vi "VisualInspection.vi"(0 "Picture Name":string, 1 "Upper":dbl, 2 "Lower":dbl, 5 "MessageIn":string) -> (3 "Message:":string, 7 "Result":string, 9 "Next Step STS":bool, 10 "Button Pressing Status":string)   [LabVIEW 2011]
panel:
  out "appended path":path
  out "LED Pressing Status":string
  in  "No Light Up On LED":bool
  in  "Light Up on LED":bool
  out "Picture:":picture
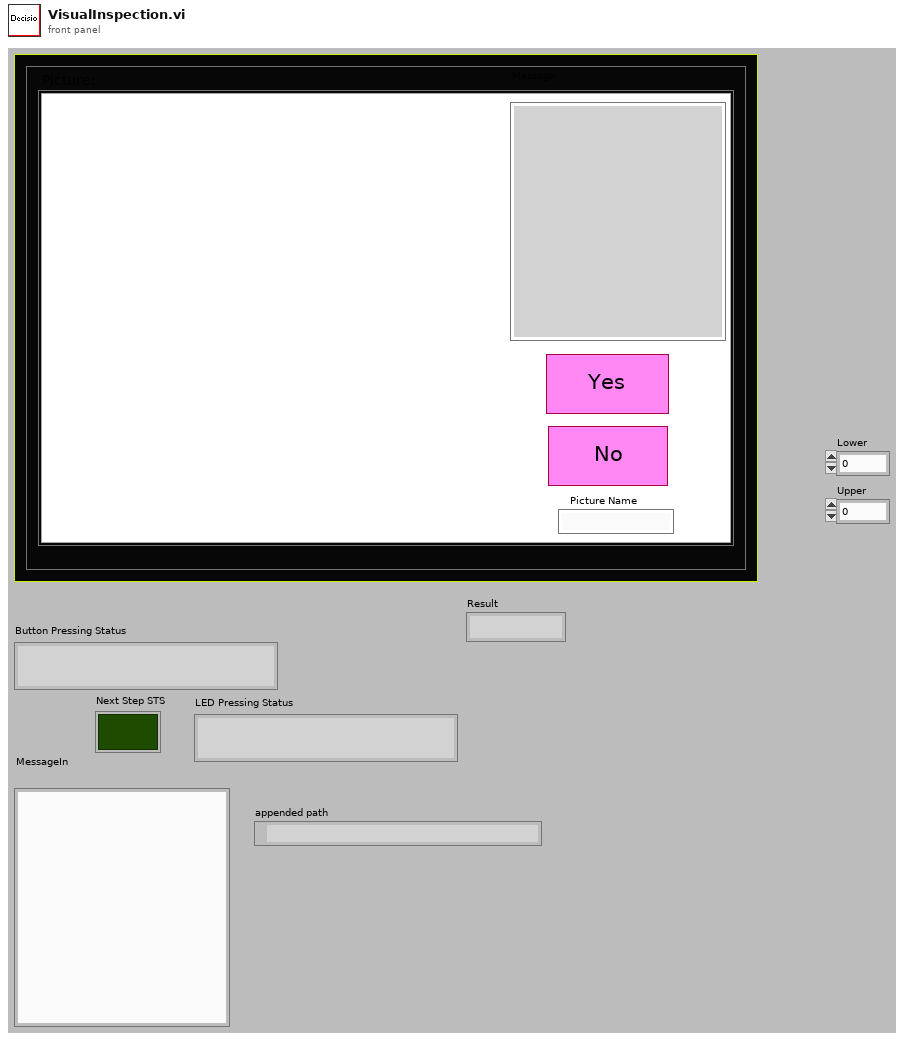
[diagram p1: front panel]
types:
  T1 = typedef "imagedata.ctl" = cluster{"image type":i32, "image depth":i32, "image":u8[], "mask":u8[], "colors":u32[], "Rectangle":cluster{"left":i16, "top":i16, "right":i16, "bottom":i16}}
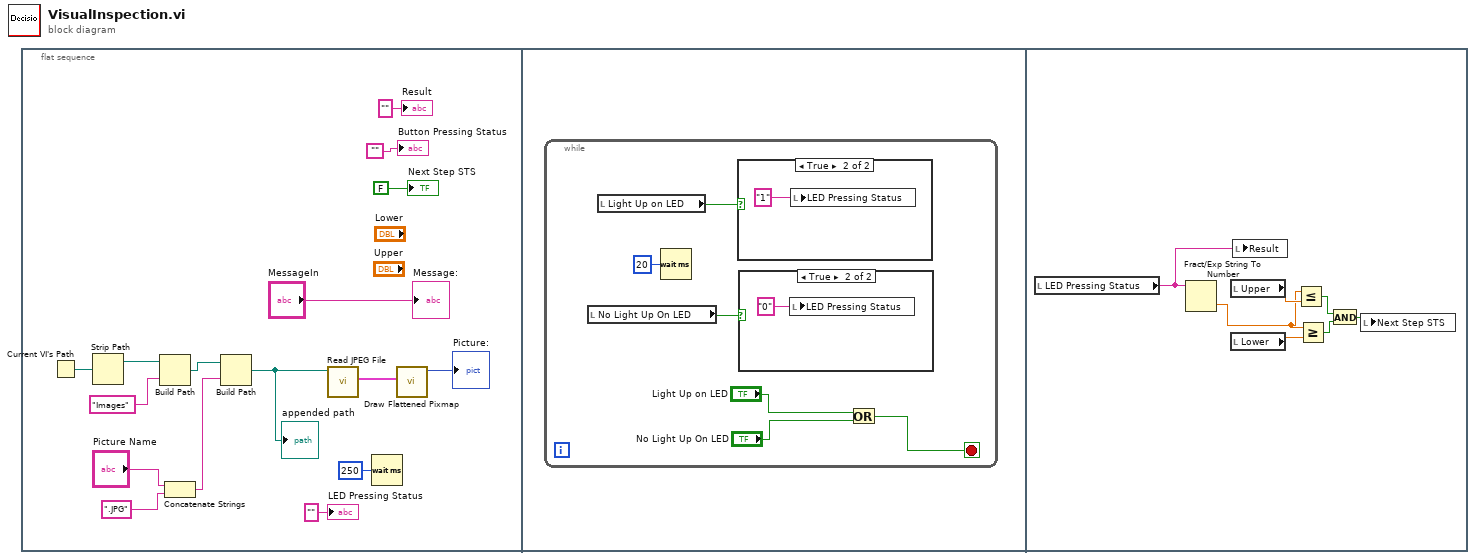
[diagram p0: block diagram]
diagram:
  n1 = flat-sequence {
    frame #0 {
      n2 = Current VI's Path() -> (path=w8:path)
      n3 = Strip Path(path=w8) -> (stripped path=w7:path)  [unwired: 1 out]
      n4 = Build Path(base path=w7, name or relative path="Images") -> (appended path=w5:path)
      n5 = Concatenate Strings("Picture Name", ".JPG" ("string")) -> (w1:string)
      n6 = Build Path(base path=w5, name or relative path=w1) -> (appended path=w4:path)
      "appended path" <- w4
      n7 = call <vilib>:"Read JPEG File.vi"("path to JPEG file"=w4) -> ("image data"=w14:T1)  [unwired: 1 in, 9 out]
      n8 = Wait (ms)(milliseconds to wait=u32 250) -> ()  [unwired: 1 out]
      n9 = call <vilib>:"Draw Flattened Pixmap.vi"("image data"=w14) -> ("new picture"=→"Picture:":picture)  [unwired: 1 in, 7 out]
      "Button Pressing Status" <- ""
      "Next Step STS" <- FALSE ("Next Step STS")
      "Result" <- "" ("Result")
      "Message:" <- "MessageIn"
      "LED Pressing Status" <- "" ("LED Pressing Status")
    }
    frame #1 {
      n10 = while {
        stop <- w20 stop-if-true
        n11 = local read "No Light Up On LED"() -> (w18:bool)
        n12 = local read "Light Up on LED"() -> (w19:bool)
        n13 = Wait (ms)(milliseconds to wait=u32 20) -> ()  [unwired: 1 out]
        n14 = case shown="True" w19 {
          frame False {
          }
          frame True {
            n15 = local write "LED Pressing Status"("1") -> ()
          }
        }
        n16 = case shown="True" w18 {
          frame False {
          }
          frame True {
            n17 = local write "LED Pressing Status"("0") -> ()
          }
        }
        n18 = Or(x="Light Up on LED", y="No Light Up On LED") -> (x .or. y?=w20:bool)
      }
    }
    frame #2 {
      n19 = local read "LED Pressing Status"() -> (w25:string)
      n20 = Fract/Exp String To Number(string=w25) -> (number=w27:dbl)  [unwired: 4 out]
      n21 = local read "Upper"() -> (w28:dbl)
      n22 = local read "Lower"() -> (w31:dbl)
      n23 = local write "Result"(w25) -> ()
      n24 = Less Or Equal?(x=w27, y=w28) -> (x <= y?=w29:bool)
      n25 = Greater Or Equal?(x=w27, y=w31) -> (x >= y?=w30:bool)
      n26 = And(x=w29, y=w30) -> (x .and. y?=w26:bool)
      n27 = local write "Next Step STS"(w26) -> ()
    }
  }
